vi "HandleDrive.vi"(7 "Deadzone":dbl=0.1, 10 "RightMotor":dbl, 11 "LeftMotor":dbl) -> (1 "Enqueue?":bool, 2 "RightMotor":dbl, 3 "LeftMotor":dbl)   [LabVIEW 2013]
doc: "Determines whether to enqueue a drive instruction. \nIf either joystick is outside the deadzone or half/straight drive is flipped, Enqueue? outputs true.\nIf the joysticks have just entered the deadzone, the motor outputs are set to 0 and Enqueue? outputs true.\nIf they are still in the deadzone (and previously were), Enqueue? outputs false."
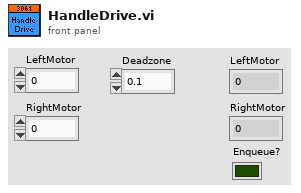
[diagram p1: front panel]
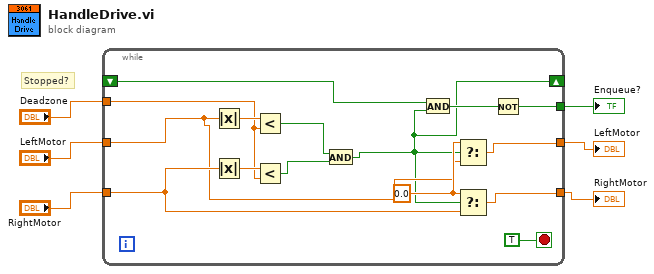
[diagram p0: block diagram]
diagram:
  # "Stopped?"
  n1 = while {
    tunnel: "LeftMotor" -> [w11]
    tunnel: "RightMotor" -> [w12]
    tunnel: "Deadzone" -> [w18]
    tunnel: [w17] -> w3
    tunnel: [w16] -> w2
    shift-right: [w7] -> _
    shift-left: _ -> [w10]
    tunnel: [w9] -> w1
    stop <- TRUE stop-if-true
    w13 = 0.0
    n2 = Absolute Value(x=w11) -> (abs(x)=w19:dbl)
    n3 = Absolute Value(x=w12) -> (abs(x)=w20:dbl)
    n4 = Less?(x=w19, y=w18) -> (x < y?=w15:bool)
    n5 = Less?(x=w20, y=w18) -> (x < y?=w14:bool)
    n6 = And(x=w15, y=w14) -> (x .and. y?=w7:bool)
    n7 = And(x=w10, y=w7) -> (x .and. y?=w8:bool)
    n8 = Select(t=w13, s=w7, f=w11) -> (s? t:f=w17:dbl)
    n9 = Select(t=w13, s=w7, f=w12) -> (s? t:f=w16:dbl)
    n10 = Not(x=w8) -> (.not. x?=w9:bool)
  }
  "Enqueue?" <- w1
  "RightMotor" <- w2
  "LeftMotor" <- w3
